vi "AutoDeposite.vi"(8 "error in (no error)":errorcluster, 9 "ClawOpenClose":bool) -> (0 "error out":errorcluster)   [LabVIEW 2020]
doc: "Auto deposite\nInputs:\n--ErrorIn--Numeric--"
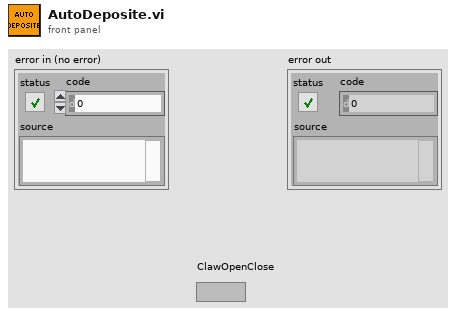
[diagram p1: front panel]
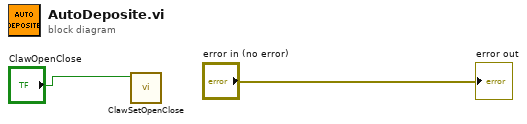
[diagram p0: block diagram]
diagram:
  n1 = call "ClawSetOpenClose.vi"("Open?"="ClawOpenClose") -> ()  [unwired: 11 in]
  "error out" <- "error in (no error)"
